vi "Agilent DMM Set Measurement Type.vi"(8 "error in (no error)":errorcluster, 10 "Measurement Type":T1, 11 "VISA Resource Name":refnum<visa-resource-name>) -> (0 "error out":errorcluster, 3 "dup VISA Resource Name":refnum<visa-resource-name>)   [LabVIEW 2011]
doc: "This VI for the HP 8753 is used to read the sweep type.\n\n0 LINEAR FREQ\n1 LOG FREQ\n2 LIST FREQ\n3 CW TIME\n4 POWER SWEEP"
uses:
  TypeDefs/Agilent DMM Measurement Type.ctl
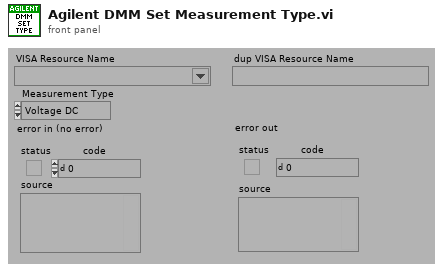
[diagram p1: front panel]
types:
  T1 = typedef "Agilent DMM Measurement Type.ctl" = enum16{"Voltage DC", "Voltage DC Ratio", "Voltage AC", "Current DC", "Current AC", "Resistance", "Fresistance", "Frequency", "Period", "Continuity", "Diode"}
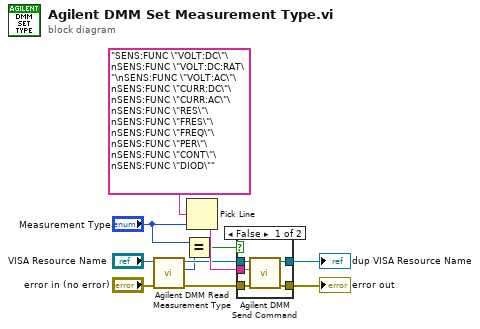
[diagram p0: block diagram]
diagram:
  n1 = call "Agilent DMM Read Measurement Type.vi"("error in (no error)"="error in (no error)", "VISA Resource Name"="VISA Resource Name") -> ("error out"=w4:errorcluster, "Measurement Type"=w3:T1, "dup VISA Resource Name"=w6:refnum<visa-resource-name>)  [unwired: 7 out]
  n2 = Equal?(x="Measurement Type", y=w3) -> (x = y?=w1:bool)
  n3 = Pick Line(multi-line string="SENS:FUNC \"VOLT:DC\"\nSENS:FUNC \"VOLT:DC:RAT\"\nSENS:FUNC \"VOLT:AC\"\nSENS:FUNC \"CURR:DC\"\nSENS:FUNC \"CURR:AC\"\nSENS:FUNC \"RES\"\nSENS:FUNC \"FRES\"\nSENS:FUNC \"FREQ\"\nSENS:FUNC \"PER\"\nSENS:FUNC \"CONT\"\nSENS:FUNC \"DIOD\"", line index="Measurement Type") -> (output string=w8:string)  [unwired: 1 out]
  n4 = case shown="False" w1 {
    tunnel: [w16 w18] -> w11
    tunnel: [w15 w17] -> w10
    tunnel: w8 -> [w14 _]
    tunnel: w6 -> [w13 w18]
    tunnel: w4 -> [w12 w17]
    frame False {
      n5 = call "Agilent DMM Send Command.vi"("error in (no error)"=w12, "Command"=w14, "VISA Resource Name"=w13) -> ("error out"=w15:errorcluster, "dup VISA Resource Name"=w16:refnum<visa-resource-name>)  [unwired: 2 in, 5 out]
    }
    frame True {
    }
  }
  "dup VISA Resource Name" <- w11
  "error out" <- w10
